vi "SVPO TDMS Write.vi"   [LabVIEW 2017]
doc: "Writes single-precision waveform or scaled array data to the specified .tdms file in a format specific to the polymorphic instance. Use this VI on embedded targets that have limited computational resources. Wire data to the <B>scaled signal [EU]</B> input to determine the polymorphic instance to use or manually select the instance."
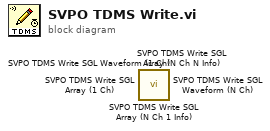
[diagram p0: block diagram]
diagram:
  n1 = call <vilib>:"SVPO TDMS Write SGL Array (N Ch 1 Info).vi"() -> ()  [unwired: 13 in, 3 out]
  n2 = call <vilib>:"SVPO TDMS Write SGL Array (N Ch N Info).vi"() -> ()  [unwired: 13 in, 3 out]
  n3 = call <vilib>:"SVPO TDMS Write SGL Array (1 Ch).vi"() -> ()  [unwired: 13 in, 3 out]
  n4 = call <vilib>:"SVPO TDMS Write SGL Waveform (N Ch).vi"() -> ()  [unwired: 13 in, 3 out]
  n5 = call <vilib>:"SVPO TDMS Write SGL Waveform (1 Ch).vi"() -> ()  [unwired: 13 in, 3 out]
